vi "SC RT.vi"() -> ()   [LabVIEW 2015]
uses:
  <vilib>/Platform/TimedLoop/XDataNode/timing_clust.ctl
  <vilib>/Platform/TimedLoop/XDataNode/nitl_modes.ctl
  <vilib>/Platform/TimedLoop/XDataNode/wakeup.ctl
  <vilib>/Platform/TimedLoop/XDataNode/loadnilvce.vi
  <vilib>/Platform/TimedLoop/XDataNode/XDataNode.xnode
  <vilib>/Platform/TimedLoop/XDataNode/XDNodeRunTimeDep.lvlib
  <vilib>/Motion/BlockNode/FB.NIMotion.xnode
  SC2 states.ctl
  <vilib>/Motion/Express/_s/nimc.fb.straightLineMove.startStraightLineMove.axis.modeRelative.0.vi
panel:
  in  "Local Encoder Offset Override":bool
  out "status":bool
  out "Encoder destination":i32
  in  "Sample equivalent to offset":i16=54
  in  "New Move":dbl format="%#_13g"
  in  "New Sample":i16
  in  "Step Window radius":i32=2
  out "Motor Done 3":bool
  out "Converted Encoder":bool[](array[boolean])
  in  "Motion Resource":refnum<k21>="Axis 1"
  out "Motor Done 2":bool
  out "Straight Line Move 2":errorcluster
  out "Raw Encoder":bool[](array[boolean])
  out "Encoder rotation":u16(graph)
  in  "Encoder Offset":i16=2790
  out "Encoder position":dbl(slide) scale=0.0..16383.0
  out "Encoder Position":i32
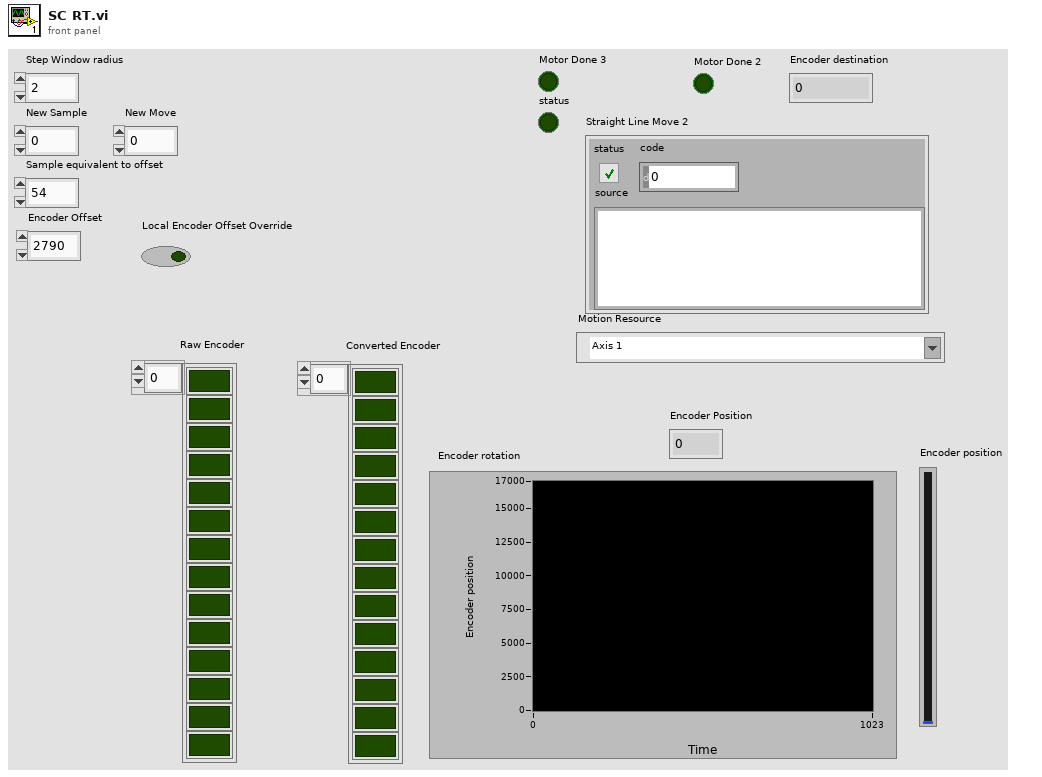
[diagram p1: front panel]
types:
  T1 = typedef "SC2 states.ctl" = enum16{"wait", "rotate wheel", "check position"}
  T2 = typedef "XDNodeRunTimeDep.lvlib/timing_clust.ctl" = cluster{"Expected End [f-1]":u64, "Actual End [f-1]":u64, "Finished Late? [f-1]":bool, "Expected End [i-1]":u64, "Actual End [i-1]":u64, "Finished Late? [i-1]":bool, "Expected Start [i]":u64, "Actual Start [i]":u64, "Expected Start [f]":u64, "Actual Start [f]":u64, "Source Name":string, "Structure Name":string, "Period":i64, "Deadline":i64, "Offset":i64, "Start":i64, "Priority":i32, "Timeout":i32, "Mode":T3, "Wakeup Reason":T4, "Error":errorcluster, "Source Type":string, "Secondary Source Type":string, "Global End Time":u64, "Global Start Time":u64, "Frame Duration":u64, "Iteration Duration":u64, "Assigned CPU":i32, "I/O Scan Engine Mode":u32}
  T3 = typedef "XDNodeRunTimeDep.lvlib/nitl_modes.ctl" = enum32{"No Change", "Process missed periods, maintain original phase", "Discard missed periods, maintain original phase", "Process missed periods, ignore original phase", "Discard missed periods, ignore original phase"}
  T4 = typedef "XDNodeRunTimeDep.lvlib/wakeup.ctl" = enum32{"Normal", "Aborted", "Asynchronous wakeup", "Timing source error", "Timed loop error", "Timeout"}
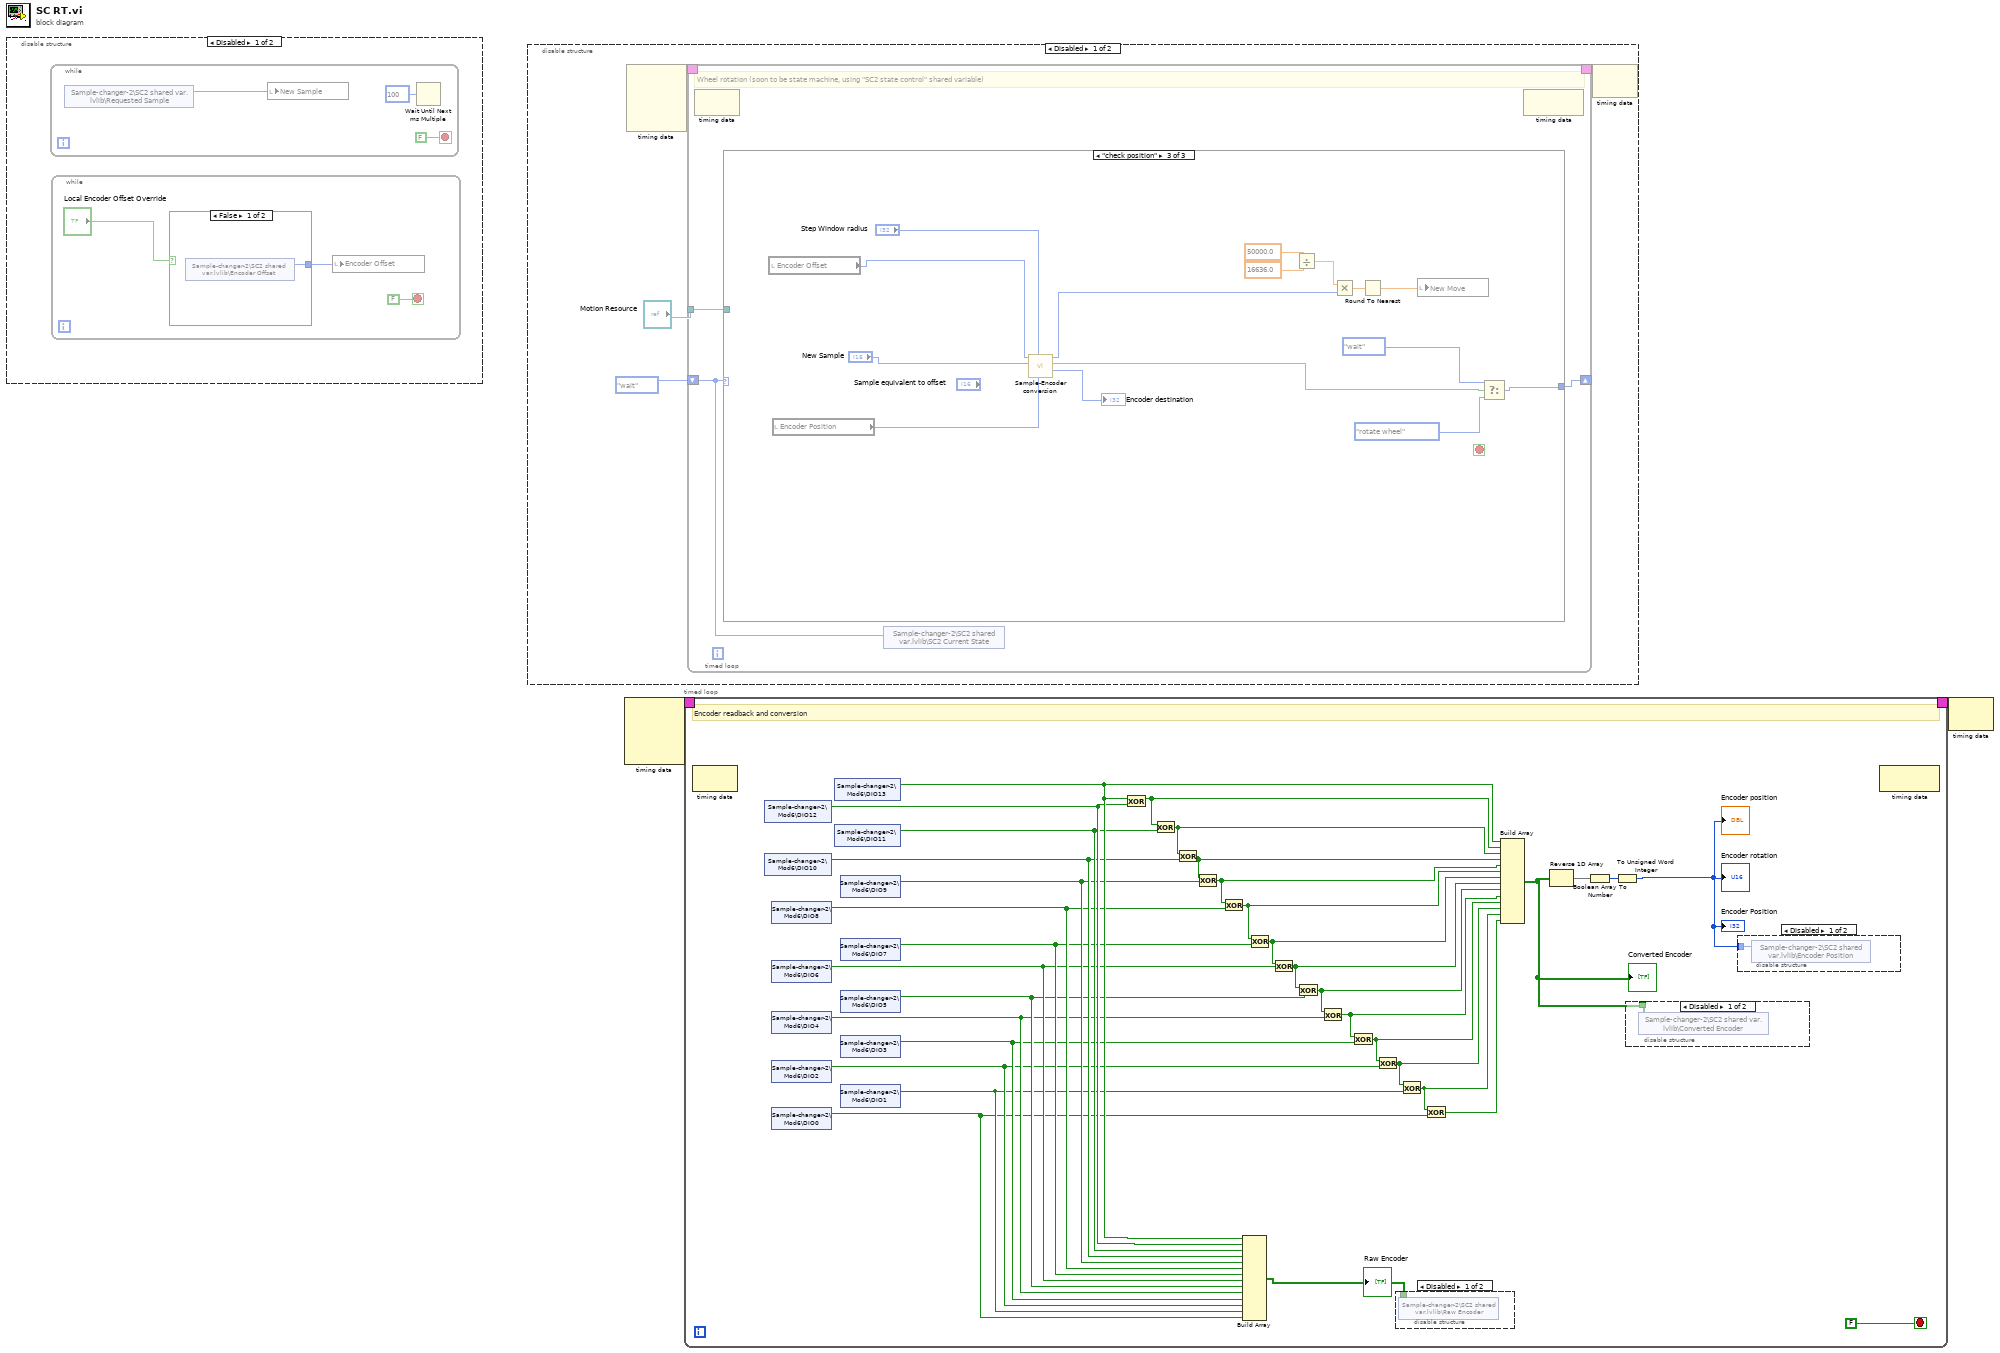
[diagram p0: block diagram]
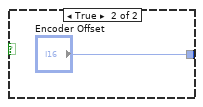
[diagram p2: hidden frame]
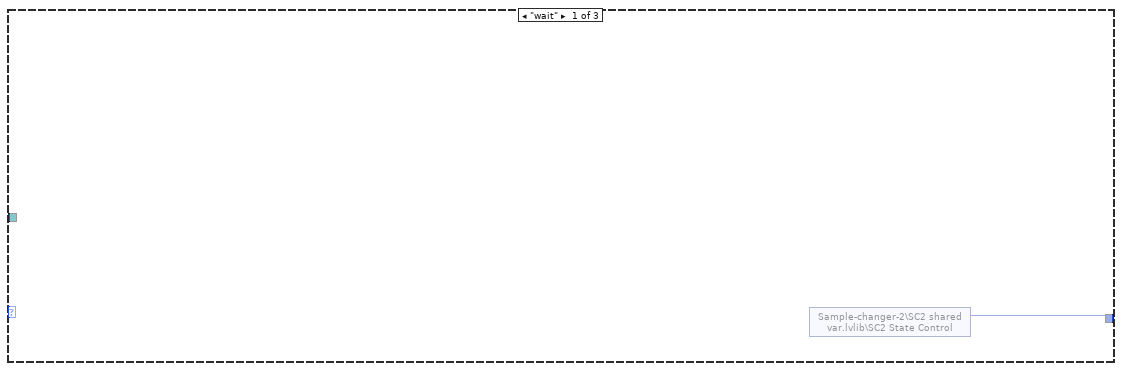
[diagram p4: hidden frame]
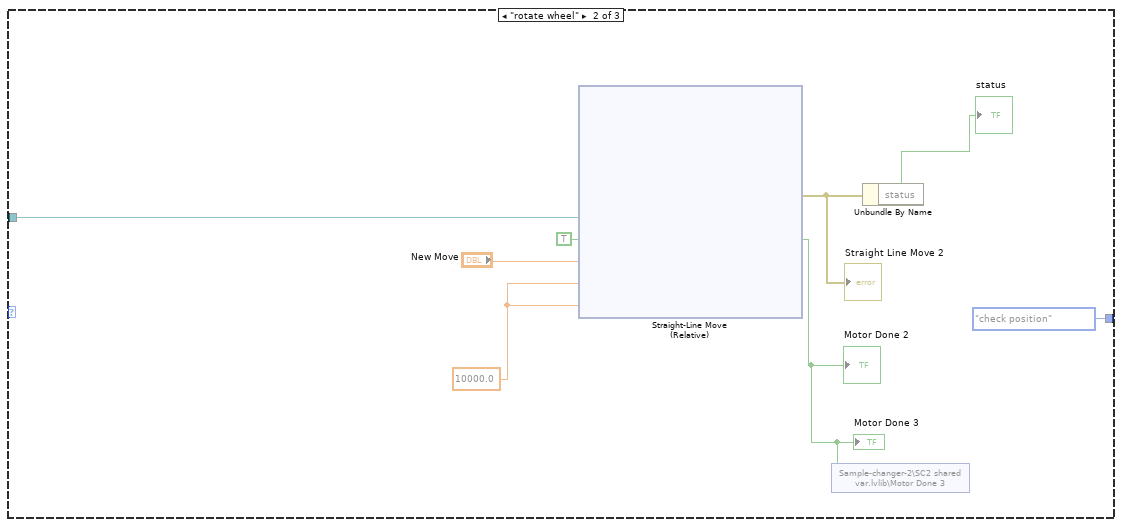
[diagram p5: hidden frame]
diagram:
  n1 = disable-structure shown="Disabled" {
    frame Disabled {
      n2 = while {
        stop <- FALSE stop-if-true
        n3 = shared-variable "Sample-changer-2\\SC2 shared var.lvlib\\Requested Sample"() -> (w9:u8)  [unwired: 1 in, 1 out]
        n4 = local write "New Sample"(w9) -> ()
        n5 = Wait Until Next ms Multiple(millisecond multiple=u32 100) -> ()  [unwired: 1 out]
      }
      n6 = while {
        stop <- FALSE stop-if-true
        n7 = case shown="False" "Local Encoder Offset Override" {
          tunnel: [w6 "Encoder Offset"] -> w4
          frame False {
            n8 = shared-variable "Sample-changer-2\\SC2 shared var.lvlib\\Encoder Offset"() -> (w6:i16)  [unwired: 1 in, 1 out]
          }
          frame True {
          }
        }
        n9 = local write "Encoder Offset"(w4) -> ()
      }
    }
    frame Enabled {
    }
  }
  n10 = disable-structure shown="Disabled" {
    frame Disabled {
      n11 = node-c288() -> (w14:T2)  [unwired: 4 in]
      n12 = timed-loop {
        tunnel: "Motion Resource" -> [w17]
        timing: w14 -> [_]
        timing-out: [_] -> w13
        shift-right: [w16] -> _
        shift-left: SC2_states."wait" -> [w15]
        stop <- _ stop-if-true
        # "Wheel rotation (soon to be state machine, using \"SC2 state control\" shared variable)"
        n13 = node-c288() -> ()  [unwired: 1 in, 1 out]
        n14 = case shown="\"check position\"" w15 {
          tunnel: w17 -> [_ w25 _]
          tunnel: [w18 SC2_states."check position" w58] -> w16
          frame "wait" {
            n15 = shared-variable "Sample-changer-2\\SC2 shared var.lvlib\\SC2 State Control"() -> (w18:T1)  [unwired: 1 in, 1 out]
          }
          frame "rotate wheel" {
            w26 = 10000.0
            n16 = xnode "Straight-Line Move\n(Relative)"("resource"=w25, "execute"=TRUE, "position"="New Move", "velocity"=w26, "acceleration"=w26) -> ("error out"=w24:errorcluster, "done"=w23:bool)  [unwired: 1 in, 1 out]
            "Straight Line Move 2" <- w24
            "Motor Done 2" <- w23
            "Motor Done 3" <- w23
            n17 = shared-variable "Sample-changer-2\\SC2 shared var.lvlib\\Motor Done 3"(w23) -> ()  [unwired: 1 in, 1 out]
            n18 = Unbundle By Name(w24) -> ("status"=→"status":bool)
          }
          frame "check position" {
            n19 = local read "Encoder Offset"() -> (w45:i16)
            n20 = local read "Encoder Position"() -> (w51:i32)
            n21 = call "Sample-Encoder conversion.vi"("Encoder Position"=w51, "Step Window radius"="Step Window radius", "New Sample Number"="New Sample", "Encoder offset"=w45) -> ("Encoder destination"=→"Encoder destination":i32, "Within Range?"=w52:bool, "Encoder distance to move"=w53:i32)  [unwired: 5 in]
            n22 = Divide(x=50000.0, y=16636.0) -> (x/y=w57:dbl)
            n23 = Multiply(x=w57, y=w53) -> (x*y=w54:dbl)
            n24 = Round To Nearest(number=w54) -> (nearest integer value=w44:dbl)
            n25 = local write "New Move"(w44) -> ()
            n26 = Select(t=SC2_states."wait", s=w52, f=SC2_states."rotate wheel") -> (s? t:f=w58:T1)
          }
        }
        n27 = shared-variable "Sample-changer-2\\SC2 shared var.lvlib\\SC2 Current State"(w15) -> ()  [unwired: 1 in, 1 out]
        n28 = node-c288() -> ()  [unwired: 1 in, 1 out]
      }
      n29 = node-c288(w13) -> ()  [unwired: 1 out]
    }
    frame Enabled {
    }
  }
  n30 = node-c288() -> (w2:T2)  [unwired: 4 in]
  n31 = timed-loop {
    timing: w2 -> [_]
    timing-out: [_] -> w1
    stop <- FALSE stop-if-true
    # "Encoder readback and conversion"
    n32 = node-c288() -> ()  [unwired: 1 in, 1 out]
    n33 = shared-variable "Sample-changer-2\\Mod6\\DIO12"() -> (w75:bool)  [unwired: 1 in, 1 out]
    n34 = shared-variable "Sample-changer-2\\Mod6\\DIO10"() -> (w73:bool)  [unwired: 1 in, 1 out]
    n35 = shared-variable "Sample-changer-2\\Mod6\\DIO8"() -> (w71:bool)  [unwired: 1 in, 1 out]
    n36 = shared-variable "Sample-changer-2\\Mod6\\DIO6"() -> (w69:bool)  [unwired: 1 in, 1 out]
    n37 = shared-variable "Sample-changer-2\\Mod6\\DIO4"() -> (w67:bool)  [unwired: 1 in, 1 out]
    n38 = shared-variable "Sample-changer-2\\Mod6\\DIO2"() -> (w65:bool)  [unwired: 1 in, 1 out]
    n39 = shared-variable "Sample-changer-2\\Mod6\\DIO0"() -> (w63:bool)  [unwired: 1 in, 1 out]
    n40 = shared-variable "Sample-changer-2\\Mod6\\DIO13"() -> (w76:bool)  [unwired: 1 in, 1 out]
    n41 = shared-variable "Sample-changer-2\\Mod6\\DIO11"() -> (w74:bool)  [unwired: 1 in, 1 out]
    n42 = shared-variable "Sample-changer-2\\Mod6\\DIO9"() -> (w72:bool)  [unwired: 1 in, 1 out]
    n43 = shared-variable "Sample-changer-2\\Mod6\\DIO7"() -> (w70:bool)  [unwired: 1 in, 1 out]
    n44 = shared-variable "Sample-changer-2\\Mod6\\DIO5"() -> (w68:bool)  [unwired: 1 in, 1 out]
    n45 = shared-variable "Sample-changer-2\\Mod6\\DIO3"() -> (w66:bool)  [unwired: 1 in, 1 out]
    n46 = shared-variable "Sample-changer-2\\Mod6\\DIO1"() -> (w64:bool)  [unwired: 1 in, 1 out]
    n47 = Exclusive Or(1:w75, 2:w76) -> (0:w80:bool)
    n48 = Exclusive Or(1:w74, 2:w80) -> (0:w94:bool)
    n49 = Exclusive Or(1:w73, 2:w94) -> (0:w93:bool)
    n50 = Exclusive Or(1:w72, 2:w93) -> (0:w92:bool)
    n51 = Exclusive Or(1:w71, 2:w92) -> (0:w91:bool)
    n52 = Build Array(w76, w75, w74, w73, w72, w71, w70, w69, w68, w67, w66, w65, w64, w63) -> (w77:bool[])
    "Raw Encoder" <- w77
    n53 = Exclusive Or(1:w70, 2:w91) -> (0:w90:bool)
    n54 = Exclusive Or(1:w69, 2:w90) -> (0:w89:bool)
    n55 = Exclusive Or(1:w68, 2:w89) -> (0:w88:bool)
    n56 = Exclusive Or(1:w67, 2:w88) -> (0:w87:bool)
    n57 = Exclusive Or(1:w66, 2:w87) -> (0:w86:bool)
    n58 = Exclusive Or(1:w65, 2:w86) -> (0:w85:bool)
    n59 = disable-structure shown="Disabled" {
      disable-tunnel: w77 -> [w96 _]
      frame Disabled {
        n60 = shared-variable "Sample-changer-2\\SC2 shared var.lvlib\\Raw Encoder"(w96) -> ()  [unwired: 1 in, 1 out]
      }
      frame Enabled {
      }
    }
    n61 = Exclusive Or(1:w64, 2:w85) -> (0:w84:bool)
    n62 = Exclusive Or(1:w63, 2:w84) -> (0:w83:bool)
    n63 = Build Array(w76, w80, w94, w93, w92, w91, w90, w89, w88, w87, w86, w85, w84, w83) -> (w79:bool[])
    "Converted Encoder" <- w79
    n64 = Reverse 1D Array(array=w79) -> (reversed array=w82:bool[])
    n65 = Boolean Array To Number(Boolean array=w82) -> (number=w81:u32)
    n66 = To Unsigned Word Integer(number=w81) -> (unsigned 16bit integer=w78:u16)
    "Encoder Position" <- w78
    "Encoder position" <- w78
    "Encoder rotation" <- w78
    n67 = disable-structure shown="Disabled" {
      disable-tunnel: w79 -> [w97 _]
      frame Disabled {
        n68 = shared-variable "Sample-changer-2\\SC2 shared var.lvlib\\Converted Encoder"(w97) -> ()  [unwired: 1 in, 1 out]
      }
      frame Enabled {
      }
    }
    n69 = disable-structure shown="Disabled" {
      disable-tunnel: w78 -> [w98 _]
      frame Disabled {
        n70 = shared-variable "Sample-changer-2\\SC2 shared var.lvlib\\Encoder Position"(w98) -> ()  [unwired: 1 in, 1 out]
      }
      frame Enabled {
      }
    }
    n71 = node-c288() -> ()  [unwired: 1 in, 1 out]
  }
  n72 = node-c288(w1) -> ()  [unwired: 1 out]
